vi "COMI DA Out.vi"(9 "volt":sgl, 10 "ch":i32, 11 "hDevice":u32) -> (2 "function return":i32, 3 "hDevice out":u32)   [LabVIEW 2017, in "Comidll.lvlib"]
doc: "int (COMI_DA_Out) (HANDLE hDevice, int ch, float volt);"
uses:
  <userlib>/Comidll/Comidll.lvlib
  <userlib>/Comidll/Comidll.dll
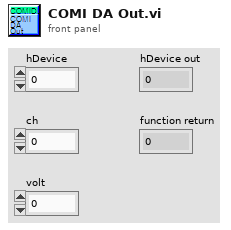
[diagram p1: front panel]
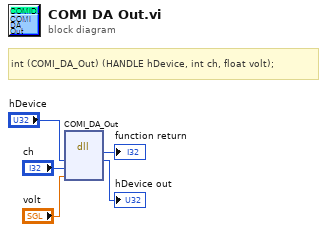
[diagram p0: block diagram]
diagram:
  # "int\t(COMI_DA_Out) (HANDLE hDevice, int ch, float volt);"
  n1 = dll-call lib="C:/Program Files/National Instruments/LabVIEW 2017/user.lib/Comidll/Comidll.*" fn="COMI_DA_Out"("hDevice"="hDevice", "ch"="ch", "volt"="volt") -> (→"function return":i32, "hDevice"=→"hDevice out":u32)  [unwired: 5 in, 2 out]
